vi "clipconf_search.vi"(0 "input cluster":T1, 1 "Channel":i32, 2 "vclip":i32, 5 "Vatt init":i32, 7 "Boolean":bool=TRUE, 9 "Voltage value":dbl=0.05, 11 "error out 2":errorcluster, 12 "Att/clip":bool=TRUE, 13 "conf value":i32=100, 14 "Delay":i32) -> (4 "output cluster":T1, 6 "Vatt init":i32, 8 "vclip":i32, 10 "L1 value":i32, 15 "error out":errorcluster)   [LabVIEW 2009]
uses:
  <vilib>/Utility/NIReport.llb/NI_report.lvclass
  <instrlib>/Agilent 81150/Agilent 81150.lvlib
panel:
  out "L1 vs vatt":cluster{i64[], i32[]}(graph)
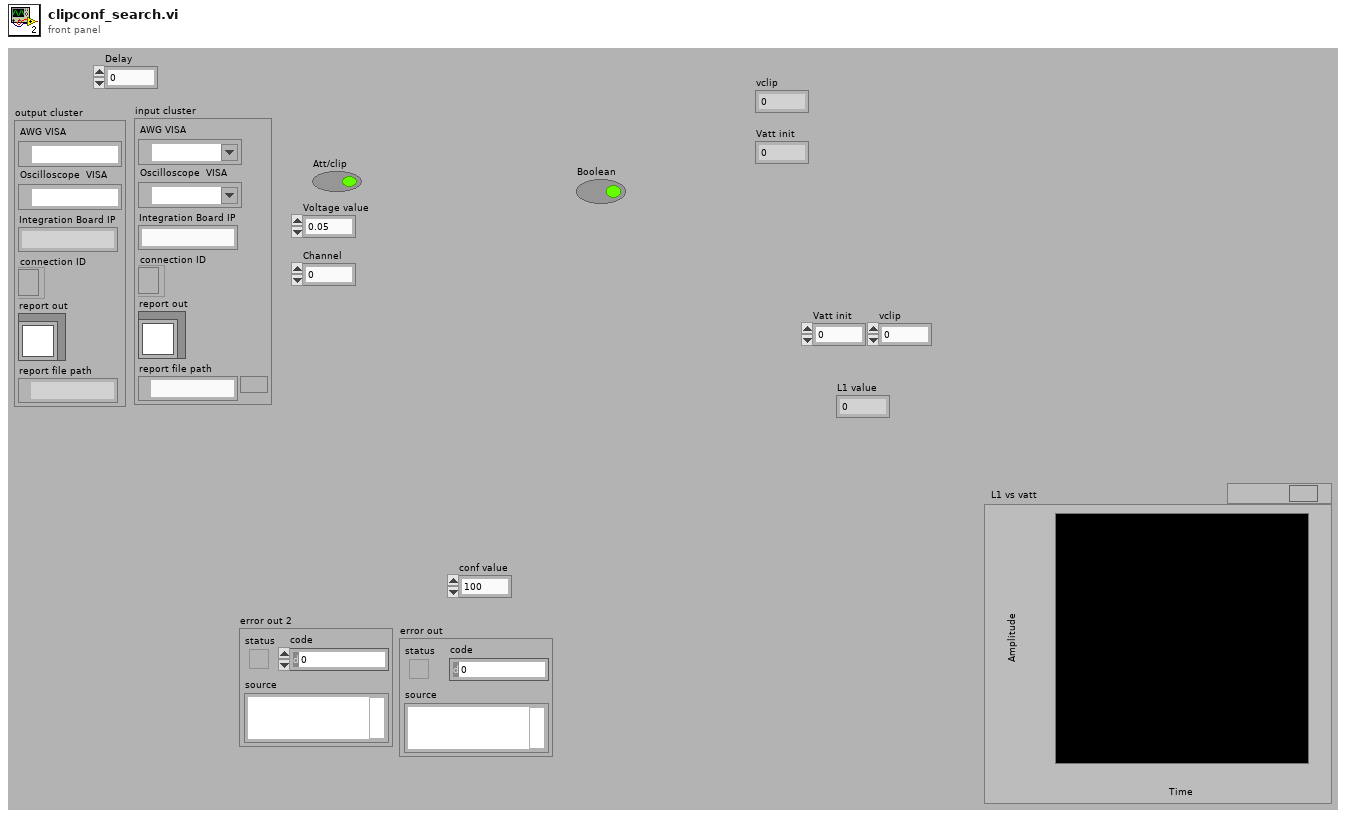
[diagram p1: front panel]
types:
  T1 = cluster{"AWG VISA":refnum<visa-resource-name>, "Oscilloscope  VISA ":refnum<visa-resource-name>, "Integration Board IP":string, "connection ID":refnum<k5>, "report out":refnum<class "NI_report.lvclass">, "report file path":path}
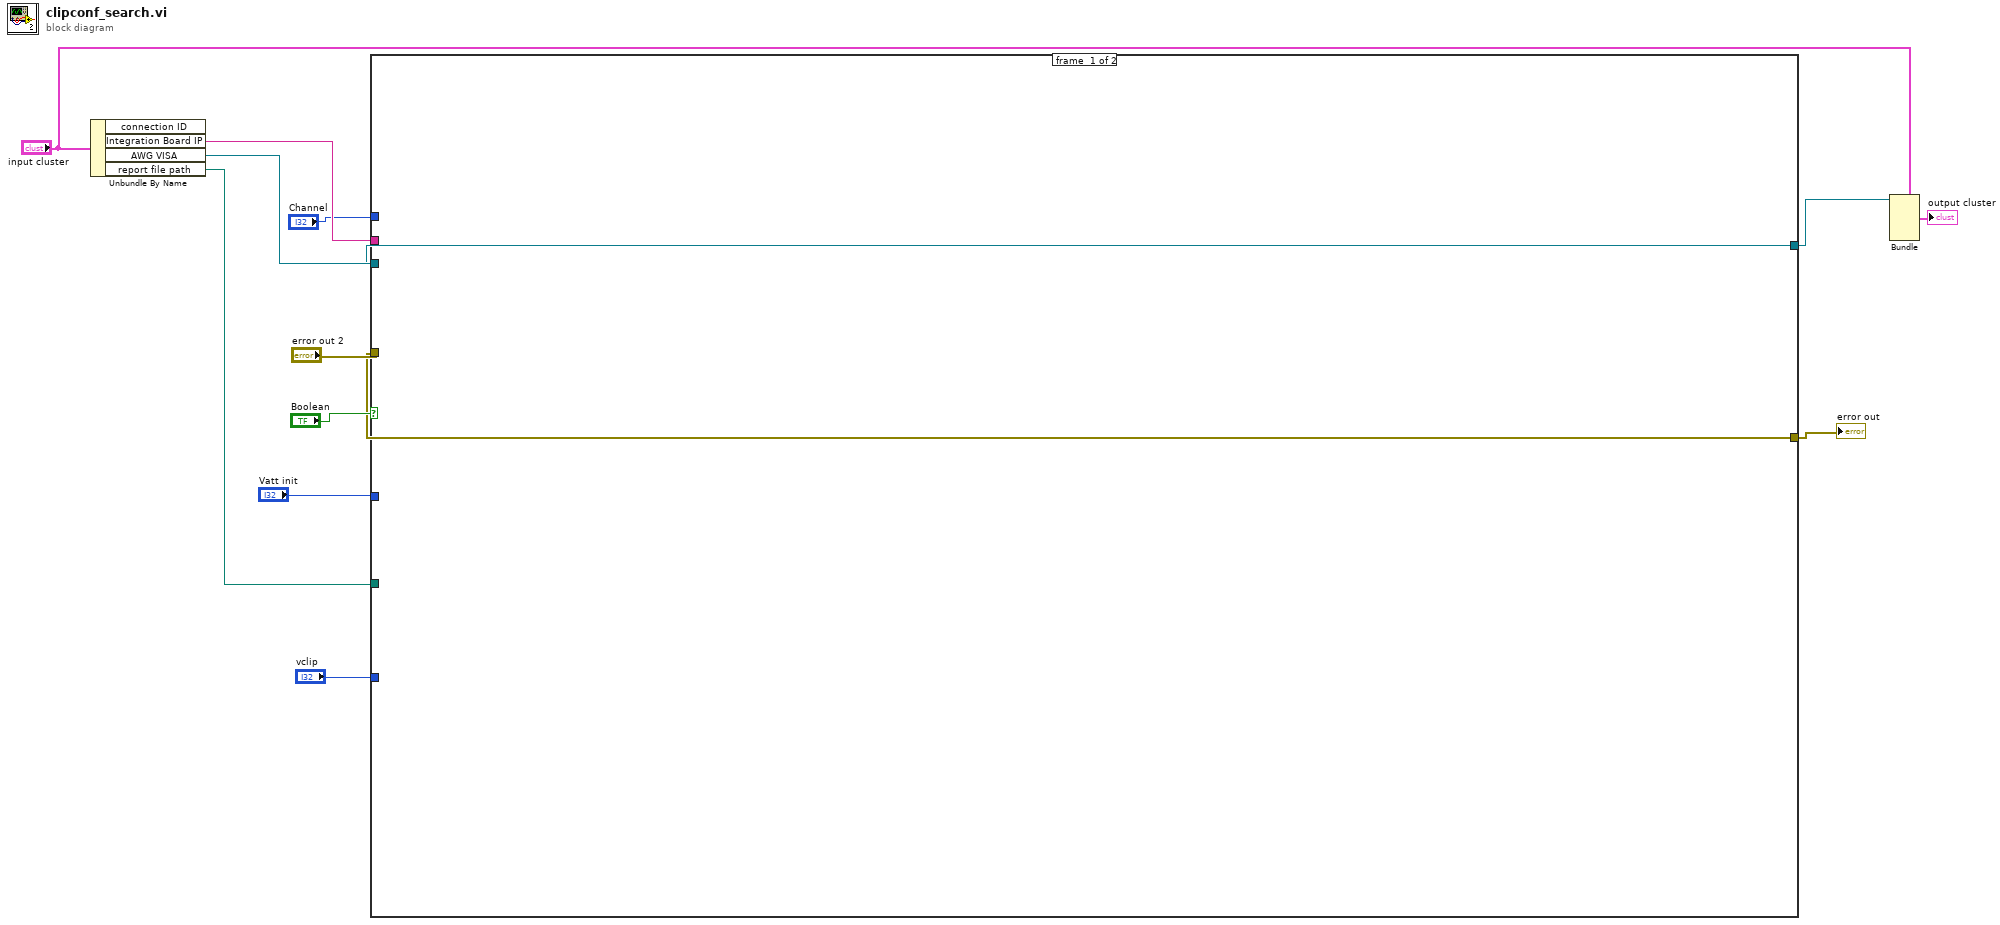
[diagram p0: block diagram]
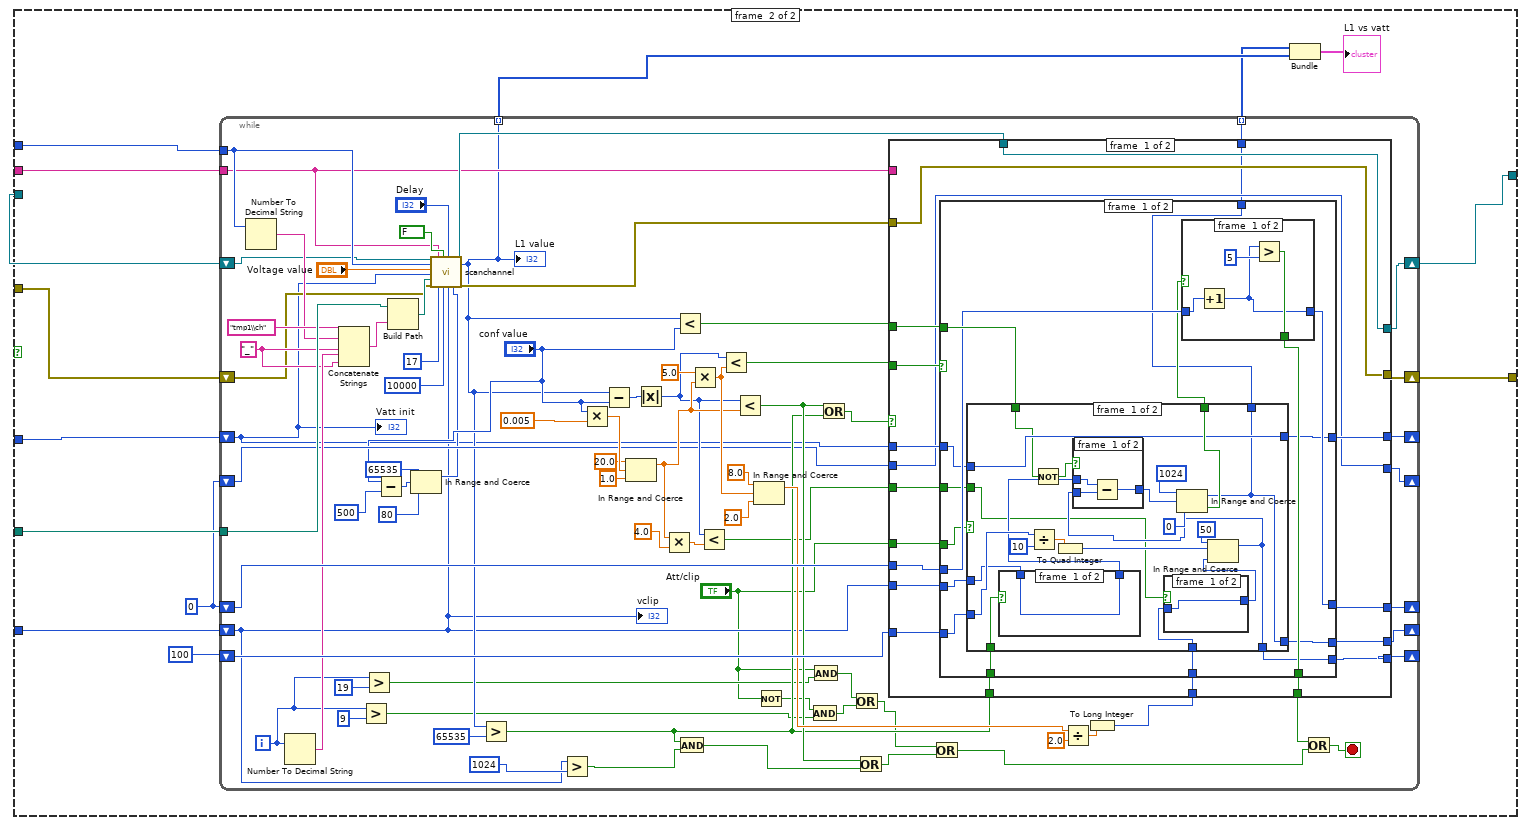
[diagram p2: hidden frame]
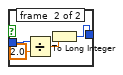
[diagram p3: hidden frame]
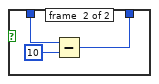
[diagram p4: hidden frame]
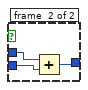
[diagram p5: hidden frame]
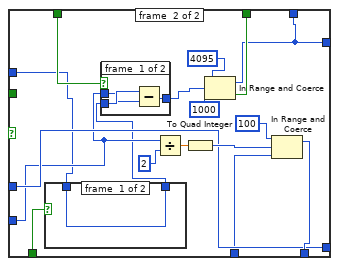
[diagram p6: hidden frame]
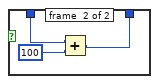
[diagram p7: hidden frame]
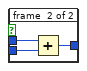
[diagram p8: hidden frame]
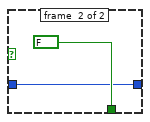
[diagram p9: hidden frame]
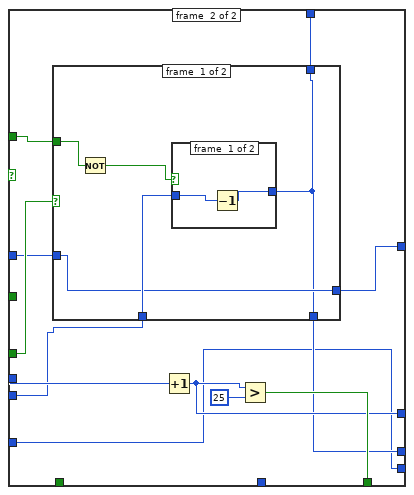
[diagram p10: hidden frame]
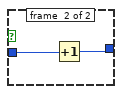
[diagram p11: hidden frame]
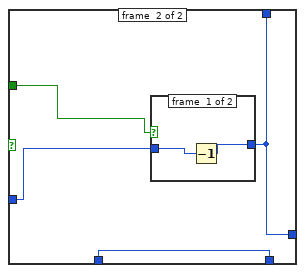
[diagram p12: hidden frame]
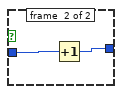
[diagram p13: hidden frame]
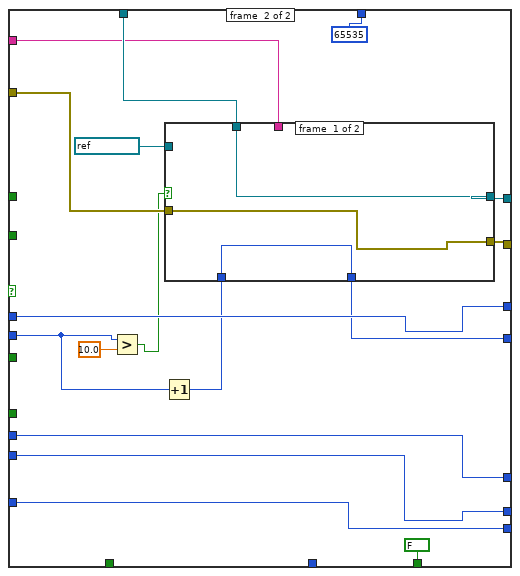
[diagram p14: hidden frame]
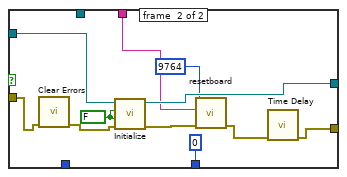
[diagram p15: hidden frame]
diagram:
  n1 = Unbundle By Name("input cluster") -> ("Integration Board IP"=w8:string, "AWG VISA"=w1:refnum<visa-resource-name>, "report file path"=w9:path)  [unwired: 1 out]
  n2 = case shown="True" "Boolean" {
    tunnel: "error out 2" -> [w14 w19]
    tunnel: w8 -> [_ w28]
    tunnel: w9 -> [_ w27]
    tunnel: "vclip" -> [_ w26]
    tunnel: "Vatt init" -> [_ w25]
    tunnel: [w14 w22] -> w12
    tunnel: "Channel" -> [_ w23]
    tunnel: [w13 w20] -> w3
    tunnel: w1 -> [w13 w21]
    frame #0 {
    }
    frame #1 {
      w18 = 0
      n3 = while {
        tunnel: w28 -> [w54]
        tunnel: w27 -> [w107]
        shift-right: [w106] -> _
        shift-left: w25 -> [w45]
        shift-right: [w86] -> _
        shift-left: w26 -> [w44]
        shift-right: [w105] -> _
        shift-left: 100 -> [w104]
        shift-right: [w103] -> _
        shift-left: w18 -> [w102]
        tunnel: w23 -> [w87]
        shift-right: [w57] -> w20
        shift-left: w21 -> [w62]
        shift-right: [w59] -> w22
        shift-left: w19 -> [w61]
        shift-right: [w55] -> _
        shift-left: w18 -> [w56]
        tunnel: [w46] -> w17 mode=indexing
        tunnel: [w43] -> w15 mode=indexing
        i -> [w42]
        stop <- w101 stop-if-true
        w88 = "_" ("string")
        n4 = Number To Decimal String(number=w87) -> (decimal integer string=w90:string)  [unwired: 1 in]
        n5 = Number To Decimal String(number=w42) -> (decimal integer string=w89:string)  [unwired: 1 in]
        n6 = Concatenate Strings("tmp1\\ch" ("name or relative path"), w90, w88, w89, w88) -> (w92:string)
        n7 = Greater?(x=w42, y=9) -> (0:w37:bool)
        n8 = Greater?(x=w42, y=19) -> (0:w39:bool)
        n9 = Subtract(x="conf value", y=500) -> (x-y=w50:i32)
        n10 = Build Path(base path=w107, name or relative path=w92) -> (appended path=w96:path)
        n11 = In Range and Coerce(upper limit=65535, x=w50, lower limit=80) -> (coerced(x)=w49:i32)  [unwired: 1 out]
        n12 = call "scanchannel.vi"("VISA resource name out"=w62, "num ch"=w87, "Voltage value"="Voltage value", "Init vatt value"=w45, "base path"=w96, "error in"=w61, "Integration Board IP"=w54, "L1 Address"=17 ("Value"), "Save test data"=FALSE, "Ch burst"=10000, "Delay"="Delay", "vclip"=w44, "initial value"=w49) -> ("VISA resource name out 2"=w58:refnum<visa-resource-name>, "L1 value"=w46:i32, "error out"=w60:errorcluster)  [unwired: 4 in]
        "L1 value" <- w46
        n13 = Greater?(x=w46, y=65535) -> (0:w65:bool)
        n14 = Greater?(x=w44, y=1024) -> (0:w64:bool)
        n15 = Multiply(x="conf value", y=0.005) -> (x*y=w78:dbl)
        n16 = Subtract(x=w46, y="conf value") -> (x-y=w99:i32)
        n17 = In Range and Coerce(upper limit=20.0, x=w78, lower limit=1.0) -> (coerced(x)=w75:dbl)  [unwired: 1 out]
        n18 = Absolute Value(x=w99) -> (abs(x)=w73:i32)
        n19 = Multiply(x=w75, y=4.0) -> (x*y=w72:dbl)
        n20 = Less?(x=w46, y="conf value") -> (x < y?=w98:bool)
        n21 = And(x=w65, y=w64) -> (x .and. y?=w63:bool)
        n22 = Multiply(x=5.0, y=w75) -> (x*y=w82:dbl)
        n23 = Less?(x=w73, y=w72) -> (x < y?=w38:bool)
        n24 = Less?(x=w73, y=w82) -> (x < y?=w97:bool)
        n25 = Less?(x=w73, y=w75) -> (x < y?=w66:bool)
        n26 = In Range and Coerce(upper limit=8.0, x=w82, lower limit=2.0) -> (coerced(x)=w69:dbl)  [unwired: 1 out]
        n27 = Not(x="Att/clip") -> (.not. x?=w36:bool)
        n28 = And(x=w36, y=w37) -> (x .and. y?=w33:bool)
        n29 = And(x="Att/clip", y=w39) -> (x .and. y?=w34:bool)
        n30 = Or(x=w66, y=w65) -> (x .or. y?=w79:bool)
        n31 = Or(x=w34, y=w33) -> (x .or. y?=w30:bool)
        n32 = Or(x=w66, y=w63) -> (x .or. y?=w32:bool)
        n33 = Or(x=w30, y=w32) -> (x .or. y?=w31:bool)
        n34 = Divide(x=w69, y=2.0) -> (x/y=w71:dbl)
        n35 = To Long Integer(number=w71) -> (32bit integer=w68:i32)
        n36 = case shown="False" w79 {
          tunnel: [w121 w253] -> w106
          tunnel: [w117 w252] -> w105
          tunnel: w104 -> [w123 w252]
          tunnel: [w118 w256] -> w103
          tunnel: w102 -> [w116 w256]
          tunnel: [w120 FALSE] -> w100
          tunnel: w98 -> [w126 _]
          tunnel: w97 -> [w122 _]
          tunnel: [w119 w255] -> w86
          tunnel: "Att/clip" -> [w125 _]
          tunnel: w65 -> [w114 _]
          tunnel: w45 -> [w115 w253]
          tunnel: w44 -> [w124 w255]
          tunnel: w68 -> [w113 _]
          tunnel: w60 -> [w111 w251]
          tunnel: [w111 w250] -> w59
          tunnel: w58 -> [w112 w248]
          tunnel: [w112 w249] -> w57
          tunnel: w56 -> [w110 w245]
          tunnel: [w110 w242] -> w55
          tunnel: w54 -> [_ w244]
          tunnel: [w109 i64 65535 ("upper limit")] -> w43
          tunnel: w38 -> [w108 _]
          frame #0 {
            n37 = case shown="False" w122 {
              tunnel: [w135 w215] -> w121
              tunnel: [w136 w212] -> w117
              tunnel: w123 -> [w142 w212]
              tunnel: [w139 w219] -> w118
              tunnel: w116 -> [w140 w222]
              tunnel: [w138 w220] -> w120
              tunnel: w126 -> [w141 w218]
              tunnel: [w134 w216] -> w119
              tunnel: w124 -> [w133 w214]
              tunnel: w125 -> [w132 w217]
              tunnel: w114 -> [w131 _]
              tunnel: w115 -> [w130 w213]
              tunnel: w113 -> [w129 _]
              tunnel: [w128 w211] -> w109
              tunnel: w108 -> [w127 _]
              frame #0 {
                n38 = case shown="False" w132 {
                  tunnel: w142 -> [w156 w182]
                  tunnel: w141 -> [w152 w189]
                  tunnel: [w157 w188] -> w137
                  tunnel: w130 -> [w154 w180]
                  tunnel: [w145 w186] -> w136
                  tunnel: [w154 w178] -> w135
                  tunnel: [w144 w184] -> w134
                  tunnel: w133 -> [w150 w184]
                  tunnel: w131 -> [w149 w183]
                  tunnel: w129 -> [w147 w179]
                  tunnel: [w144 w178] -> w128
                  tunnel: w127 -> [w143 _]
                  frame #0 {
                    n39 = case shown="False" w149 {
                      tunnel: [w168 w170] -> w151
                      tunnel: w150 -> [w168 w171]
                      frame #0 {
                      }
                      frame #1 {
                        n40 = Subtract(x=w171, y=i64 10) -> (x-y=w170:i64)
                      }
                    }
                    n41 = Divide(x=w156, y=10) -> (x/y=w161:dbl)
                    n42 = Not(x=w152) -> (.not. x?=w153:bool)
                    n43 = To Quad Integer(1:w161) -> (0:w146:i64)
                    n44 = case shown="False" w143 {
                      tunnel: [w163 w166] -> w148
                      tunnel: w147 -> [w163 w164]
                      frame #0 {
                      }
                      frame #1 {
                        n45 = Divide(x=w164, y=2.0) -> (x/y=w167:dbl)
                        n46 = To Long Integer(number=w167) -> (32bit integer=w166:i32)
                      }
                    }
                    n47 = In Range and Coerce(upper limit=i64 50, x=w146, lower limit=w148) -> (coerced(x)=w145:i64)  [unwired: 1 out]
                    n48 = case shown="True" w153 {
                      tunnel: w151 -> [w174 w177]
                      tunnel: w145 -> [w173 w176]
                      tunnel: [w172 w175] -> w155
                      frame #0 {
                        n49 = Subtract(x=w174, y=w173) -> (x-y=w172:i64)
                      }
                      frame #1 {
                        n50 = Add(x=w177, y=w176) -> (x+y=w175:i64)
                      }
                    }
                    n51 = In Range and Coerce(upper limit=i64 1024, x=w155, lower limit=i64 0 ("upper limit")) -> (coerced(x)=w144:i64, In Range?=w157:bool)
                  }
                  frame #1 {
                    n52 = case shown="False" w183 {
                      tunnel: [w195 w198] -> w181
                      tunnel: w180 -> [w195 w197]
                      frame #0 {
                      }
                      frame #1 {
                        n53 = Add(x=w197, y=i64 100) -> (x+y=w198:i64)
                      }
                    }
                    n54 = case shown="True" w189 {
                      tunnel: w181 -> [w201 w204]
                      tunnel: w182 -> [w200 w203]
                      tunnel: [w199 w202] -> w192
                      frame #0 {
                        n55 = Subtract(x=w201, y=w200) -> (x-y=w199:i64)
                      }
                      frame #1 {
                        n56 = Add(x=w203, y=w204) -> (x+y=w202:i64)
                      }
                    }
                    n57 = Divide(x=w182, y=2) -> (x/y=w193:dbl)
                    n58 = To Quad Integer(1:w193) -> (0:w187:i64)
                    n59 = In Range and Coerce(upper limit=i64 4095, x=w192, lower limit=i64 1000 ("upper limit")) -> (coerced(x)=w178:i64, In Range?=w188:bool)
                    n60 = In Range and Coerce(upper limit=i64 100, x=w187, lower limit=w179) -> (coerced(x)=w186:i64)  [unwired: 1 out]
                  }
                }
                n61 = case shown="True" w137 {
                  tunnel: w140 -> [w206 w209]
                  tunnel: [w205 w209] -> w139
                  tunnel: [w207 FALSE] -> w138
                  frame #0 {
                    n62 = Increment(x=w206) -> (x+1=w205:i32)
                    n63 = Greater?(x=w205, y=5) -> (0:w207:bool)
                  }
                  frame #1 {
                  }
                }
              }
              frame #1 {
                n64 = case shown="True" w217 {
                  tunnel: w214 -> [w226 w234]
                  tunnel: [w223 w234] -> w216
                  tunnel: w218 -> [w225 w235]
                  tunnel: [w224 w232] -> w215
                  tunnel: w213 -> [w224 w233]
                  tunnel: [w223 w232] -> w211
                  frame #0 {
                    n65 = Not(x=w225) -> (.not. x?=w227:bool)
                    n66 = case shown="True" w227 {
                      tunnel: w226 -> [w228 w231]
                      tunnel: [w229 w230] -> w223
                      frame #0 {
                        n67 = Decrement(x=w228) -> (x-1=w229:i64)
                      }
                      frame #1 {
                        n68 = Increment(x=w231) -> (x+1=w230:i64)
                      }
                    }
                  }
                  frame #1 {
                    n69 = case shown="True" w235 {
                      tunnel: w233 -> [w236 w239]
                      tunnel: [w237 w238] -> w232
                      frame #0 {
                        n70 = Decrement(x=w236) -> (x-1=w237:i64)
                      }
                      frame #1 {
                        n71 = Increment(x=w239) -> (x+1=w238:i64)
                      }
                    }
                  }
                }
                n72 = Increment(x=w222) -> (x+1=w219:i32)
                n73 = Greater?(x=w219, y=25) -> (0:w220:bool)
              }
            }
          }
          frame #1 {
            n74 = Greater?(x=w245, y=10.0) -> (0:w246:bool)
            n75 = Increment(x=w245) -> (x+1=w243:i32)
            n76 = case shown="False" w246 {
              tunnel: w251 -> [w258 w262]
              tunnel: [w258 w266] -> w250
              tunnel: [w259 w270] -> w249
              tunnel: w248 -> [w259 _]
              tunnel: w244 -> [_ w264]
              tunnel: [w257 0] -> w242
              tunnel: w243 -> [w257 _]
              tunnel: refnum<visa-resource-name> "81160A" ("VISA resource name") -> [_ w260]
              frame #0 {
              }
              frame #1 {
                w269 = FALSE ("Reset (True)")
                n77 = call <vilib>:"Clear Errors.vi"("error in (no error)"=w262) -> ("error out"=w261:errorcluster)  [unwired: 6 in]
                n78 = call <instrlib>:"Initialize.vi"("error in (no error)"=w261, "Reset (True)"=w269, "ID Query (True)"=w269, "VISA resource name"=w260) -> ("error out"=w268:errorcluster, "VISA resource name out"=w270:refnum<visa-resource-name>)  [unwired: 6 in]
                n79 = call "resetboard.vi"("error in (no error)"=w268, "address"=w264, "remote port or service name"=u16 9764) -> ("error out"=w267:errorcluster)  [unwired: 7 in, 1 out]
                n80 = call "Time Delay"("error in (no error)"=w267) -> ("error out"=w266:errorcluster)  [unwired: 10 in]
              }
            }
          }
        }
        n81 = Or(x=w100, y=w31) -> (x .or. y?=w101:bool)
        "vclip" <- w44
        "Vatt init" <- w45
      }
      n82 = Bundle(w15, w17) -> (→"L1 vs vatt":cluster{i64[], i32[]})  [unwired: 1 in]
    }
  }
  "error out" <- w12
  n83 = Bundle(cluster="input cluster", "AWG VISA"=w3) -> (→"output cluster":T1)  [unwired: 5 in]
